vi "Handle Update App.vi"(7 "Sort Order":T1, 8 "error in (no error)":errorcluster, 10 "ViaApp":refnum<class "ViaApp.lvclass">, 11 "AppListPanel in":refnum<class "AppListPanel.lvclass">) -> (0 "error out":errorcluster, 3 "AppListPanel out":refnum<class "AppListPanel.lvclass">)   [LabVIEW 2020, in "PicoG-App.lvlib" / "AppListPanel.lvclass"]
uses:
  AppListPanel.lvclass
  ViaApp/ViaApp.lvclass
  AppListPanel.lvclass/AppListPanel.ctl
  Sort Order.ctl
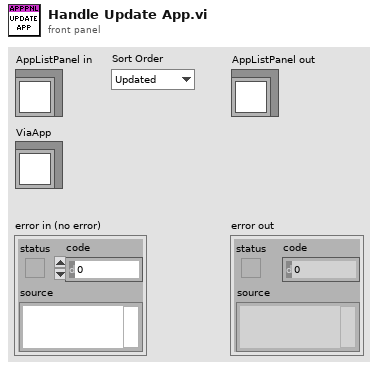
[diagram p1: front panel]
types:
  T1 = typedef "PicoG-App.lvlib/AppListPanel.lvclass/Sort Order.ctl" = enum16{"Updated", "Name"}
  T2 = typedef "PicoG-App.lvlib/AppListPanel.lvclass/Ref Data.ctl" = cluster{"App Map":map{path, refnum<class "ViaApp.lvclass">}}
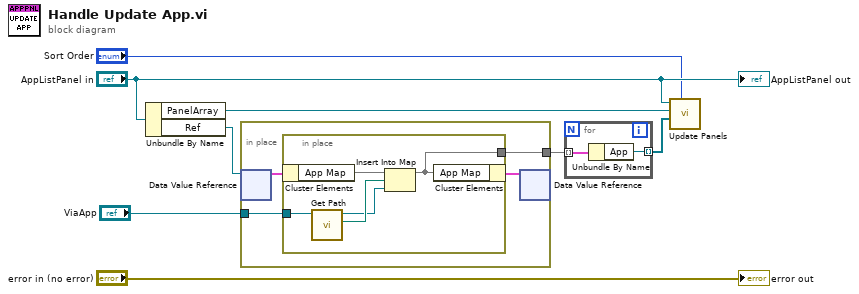
[diagram p0: block diagram]
diagram:
  n1 = Unbundle By Name("AppListPanel in") -> ("PanelArray"=w3:refnum<class "ArrayManager.lvclass">, "Ref"=w7:refnum<data-value>)
  n2 = in-place {
    in-place-border: "ViaApp" -> [w10]
    in-place-border: [w9] -> w5
    n3 = in-place-dvr #1(w7) -> (w12:T2)  [unwired: 1 out]
    n4 = in-place {
      in-place-border: w10 -> [w16]
      in-place-border: [w13] -> w9
      n5 = in-place-cluster #2(w12) -> ("App Map"=w17:map{path, refnum<class "ViaApp.lvclass">})
      n6 = call "Get Path.vi"("ViaApp in"=w16) -> ("Path"=w15:path, "ViaApp out"=w14:refnum<class "ViaApp.lvclass">)  [unwired: 8 in, 1 out]
      n7 = Insert Into Map(map in=w17, key=w15, value=w14) -> (map out=w13:map{path, refnum<class "ViaApp.lvclass">})  [unwired: 2 out]
      n8 = in-place-cluster #2("App Map"=w13) -> (w11:T2)
    }
    n9 = in-place-dvr #1(w11) -> ()  [unwired: 2 out]
  }
  n10 = for {
    tunnel: w5 -> [w19] mode=indexing
    tunnel: [w18] -> w4 mode=indexing
    n11 = Unbundle By Name(w19) -> ("App"=w18:refnum<class "ViaApp.lvclass">)
  }
  n12 = call "Update Panels.vi"("Sort Order"="Sort Order", "Apps"=w4, "PanelArray"=w3, "AppListPanel"="AppListPanel in") -> ()  [unwired: 8 in]
  "error out" <- "error in (no error)"
  "AppListPanel out" <- "AppListPanel in"
